vi "Create Events.vi"(8 "error in (no error)":errorcluster, 11 "Process State Data in":refnum<class "Process State Data.lvclass">) -> (0 "error out":errorcluster, 3 "Process State Data out":refnum<class "Process State Data.lvclass">)   [LabVIEW 2022 SP3, in "Process State Data.lvclass"]
uses:
  Process State Data.lvclass
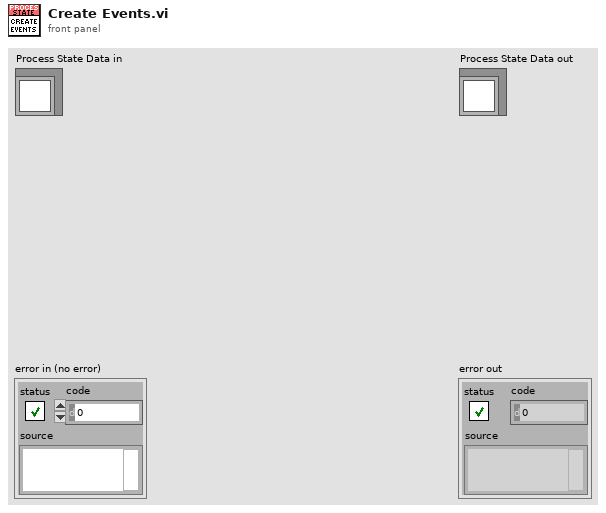
[diagram p1: front panel]
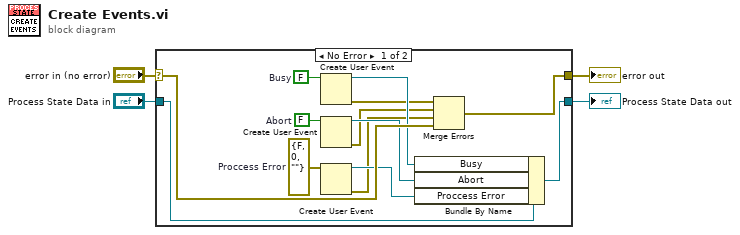
[diagram p0: block diagram]
diagram:
  n1 = case shown="No Error" "error in (no error)" {
    selector: "error in (no error)" -> [w16 w19]
    tunnel: [w8 w19] -> w3
    tunnel: [w12 w18] -> w1
    tunnel: "Process State Data in" -> [w17 w18]
    frame No Error {
      w13 = errorcluster {"status"=FALSE, "code"=0, "source"=""}  # Proccess Error
      w15 = FALSE  # Busy
      w14 = FALSE  # Abort
      n2 = Create User Event(user event datatype=w15) -> (user event=w11:refnum<user-event>, error out=w7:errorcluster)  [unwired: 1 in]
      n3 = Create User Event(user event datatype=w14) -> (user event=w10:refnum<user-event>, error out=w6:errorcluster)  [unwired: 1 in]
      n4 = Create User Event(user event datatype=w13) -> (user event=w9:refnum<user-event>, error out=w5:errorcluster)  [unwired: 1 in]
      n5 = Bundle By Name(cluster=w17, "Busy"=w11, "Abort"=w10, "Proccess Error"=w9) -> (w12:refnum<class "Process State Data.lvclass">)
      n6 = Merge Errors(w7, w6, w5, w16) -> (w8:errorcluster)
    }
    frame Error {
    }
  }
  "error out" <- w3
  "Process State Data out" <- w1
